vi "1-at-a-time.vi"(8 "error in (no error)":errorcluster, 10 "write buffer":string, 11 "VISA resource name":refnum<visa-resource-name>) -> (0 "error out":errorcluster, 3 "VISA resource name out":refnum<visa-resource-name>)   [LabVIEW 2017]
doc: "For Instruments that require characters to be written one at a time. It breaks down the string into individual bytes and transfers one at a time."
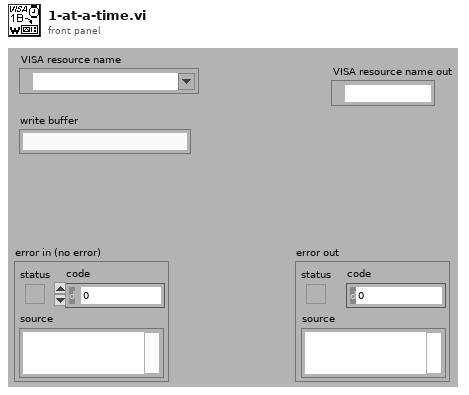
[diagram p1: front panel]
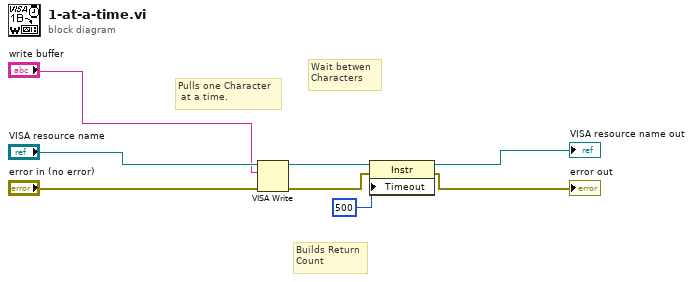
[diagram p0: block diagram]
diagram:
  # "Wait betwen \nCharacters"
  # "Builds Return\nCount"
  # "Pulls one Character\n at a time."
  n1 = VISA Write(VISA resource name="VISA resource name", write buffer="write buffer", error in (no error)="error in (no error)") -> (VISA resource name out=w3:refnum<visa-resource-name>, error out=w2:errorcluster)  [unwired: 1 out]
  n2 = property class="Instr"(reference=w3, error in=w2, "Timeout"=u32 500 ("General Settings:Timeout Value")) -> (reference out=→"VISA resource name out":refnum<visa-resource-name>, error out=→"error out":errorcluster)
